vi "DriveNetwork.vi"   [LabVIEW 2020]
uses:
  DriveGlobals.vi
  <vilib>/Rock Robotics/Network Tables/NT Write Number.vi
  <vilib>/Rock Robotics/Network Tables/NT Read Number.vi
  <vilib>/Rock Robotics/Network Tables/NT Write Boolean.vi
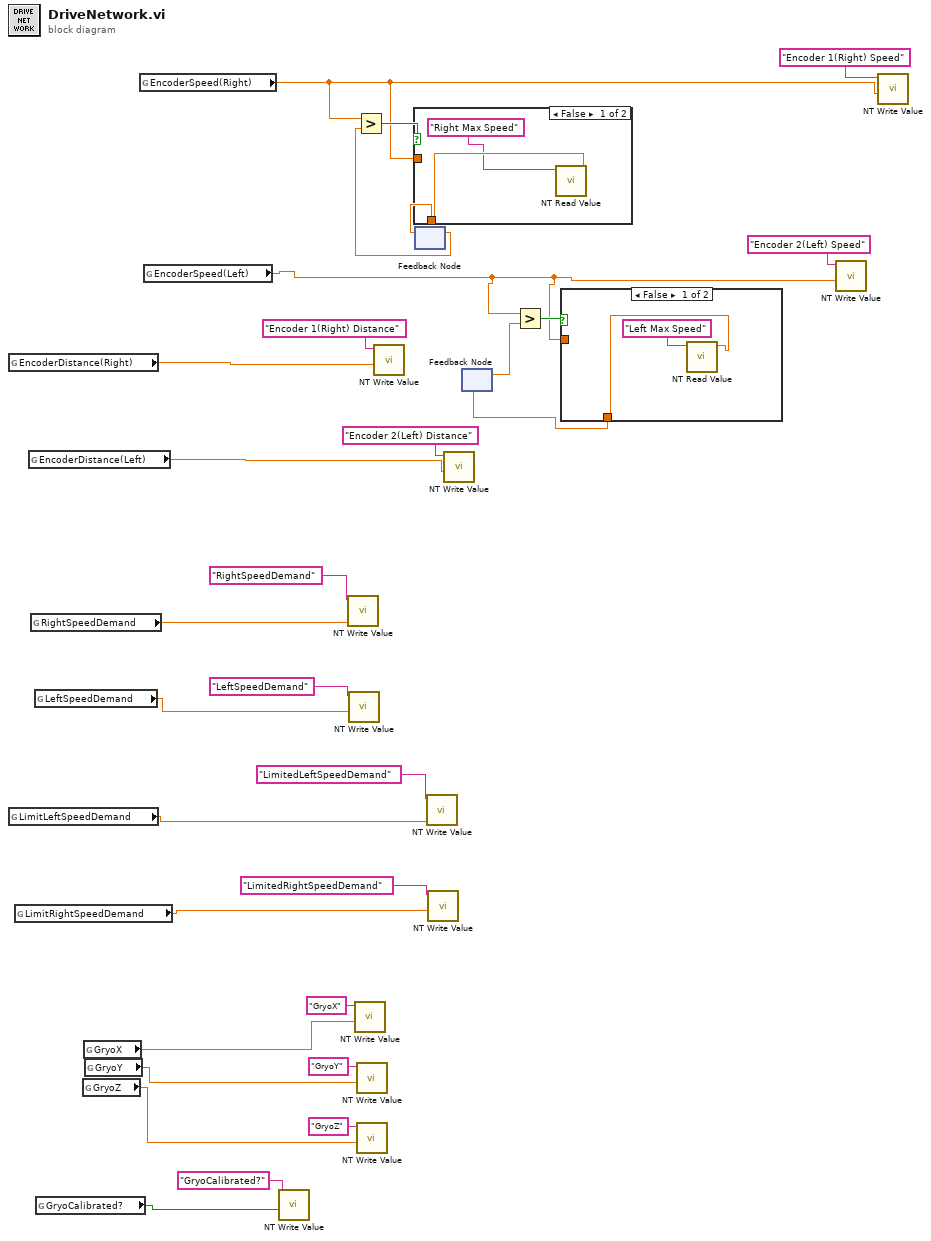
[diagram p0: block diagram]
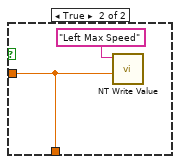
[diagram p2: hidden frame]
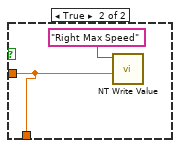
[diagram p3: hidden frame]
diagram:
  n1 = global read "DriveGlobals.vi" "EncoderDistance(Right)"() -> (w11:dbl)
  n2 = global read "DriveGlobals.vi" "LimitLeftSpeedDemand"() -> (w19:dbl)
  n3 = global read "DriveGlobals.vi" "LimitRightSpeedDemand"() -> (w20:dbl)
  n4 = global read "DriveGlobals.vi" "EncoderDistance(Left)"() -> (w12:dbl)
  n5 = global read "DriveGlobals.vi" "RightSpeedDemand"() -> (w26:dbl)
  n6 = global read "DriveGlobals.vi" "LeftSpeedDemand"() -> (w25:dbl)
  n7 = global read "DriveGlobals.vi" "GryoCalibrated?"() -> (w2:bool)
  n8 = global read "DriveGlobals.vi" "GryoZ"() -> (w3:dbl)
  n9 = global read "DriveGlobals.vi" "GryoX"() -> (w5:dbl)
  n10 = global read "DriveGlobals.vi" "GryoY"() -> (w4:dbl)
  n11 = global read "DriveGlobals.vi" "EncoderSpeed(Right)"() -> (w10:dbl)
  n12 = global read "DriveGlobals.vi" "EncoderSpeed(Left)"() -> (w9:dbl)
  n13 = call-poly <vilib>:"NT Write Value.vi"("Boolean"=w2, "Name"="GryoCalibrated?") -> ()  [unwired: 9 in, 1 out]
  n14 = call-poly <vilib>:"NT Write Value.vi"("Numeric"=w26, "Name"="RightSpeedDemand") -> ()  [unwired: 9 in, 1 out]
  n15 = call-poly <vilib>:"NT Write Value.vi"("Numeric"=w25, "Name"="LeftSpeedDemand") -> ()  [unwired: 9 in, 1 out]
  n16 = call-poly <vilib>:"NT Write Value.vi"("Numeric"=w5, "Name"="GryoX") -> ()  [unwired: 9 in, 1 out]
  n17 = call-poly <vilib>:"NT Write Value.vi"("Numeric"=w4, "Name"="GryoY") -> ()  [unwired: 9 in, 1 out]
  n18 = call-poly <vilib>:"NT Write Value.vi"("Numeric"=w3, "Name"="GryoZ") -> ()  [unwired: 9 in, 1 out]
  n19 = call-poly <vilib>:"NT Write Value.vi"("Numeric"=w11, "Name"="Encoder 1(Right) Distance") -> ()  [unwired: 9 in, 1 out]
  n20 = feedback #1() -> (w15:dbl)  [unwired: 1 in]
  n21 = Greater?(x=w10, y=w15) -> (0:w18:bool)
  n22 = case shown="False" w18 {
    tunnel: w10 -> [_ w33]
    tunnel: [w32 w33] -> w16
    frame False {
      n23 = call-poly <vilib>:"NT Read Value.vi"("Name"="Right Max Speed") -> ("Numeric"=w32:dbl)  [unwired: 9 in, 1 out]
    }
    frame True {
      n24 = call-poly <vilib>:"NT Write Value.vi"("Numeric"=w33, "Name"="Right Max Speed") -> ()  [unwired: 9 in, 1 out]
    }
  }
  n25 = feedback-in #1(w16) -> ()
  n26 = call-poly <vilib>:"NT Write Value.vi"("Numeric"=w19, "Name"="LimitedLeftSpeedDemand") -> ()  [unwired: 9 in, 1 out]
  n27 = call-poly <vilib>:"NT Write Value.vi"("Numeric"=w20, "Name"="LimitedRightSpeedDemand") -> ()  [unwired: 9 in, 1 out]
  n28 = call-poly <vilib>:"NT Write Value.vi"("Numeric"=w12, "Name"="Encoder 2(Left) Distance") -> ()  [unwired: 9 in, 1 out]
  n29 = feedback #2() -> (w13:dbl)  [unwired: 1 in]
  n30 = Greater?(x=w9, y=w13) -> (0:w17:bool)
  n31 = case shown="False" w17 {
    tunnel: w9 -> [_ w37]
    tunnel: [w36 w37] -> w14
    frame False {
      n32 = call-poly <vilib>:"NT Read Value.vi"("Name"="Left Max Speed") -> ("Numeric"=w36:dbl)  [unwired: 9 in, 1 out]
    }
    frame True {
      n33 = call-poly <vilib>:"NT Write Value.vi"("Numeric"=w37, "Name"="Left Max Speed") -> ()  [unwired: 9 in, 1 out]
    }
  }
  n34 = feedback-in #2(w14) -> ()
  n35 = call-poly <vilib>:"NT Write Value.vi"("Numeric"=w9, "Name"="Encoder 2(Left) Speed") -> ()  [unwired: 9 in, 1 out]
  n36 = call-poly <vilib>:"NT Write Value.vi"("Numeric"=w10, "Name"="Encoder 1(Right) Speed") -> ()  [unwired: 9 in, 1 out]
